vi "activeXexample.vi"() -> ()   [LabVIEW 2017]
panel:
  out "ID":i32
  out "Acq":i32
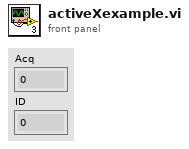
[diagram p1: front panel]
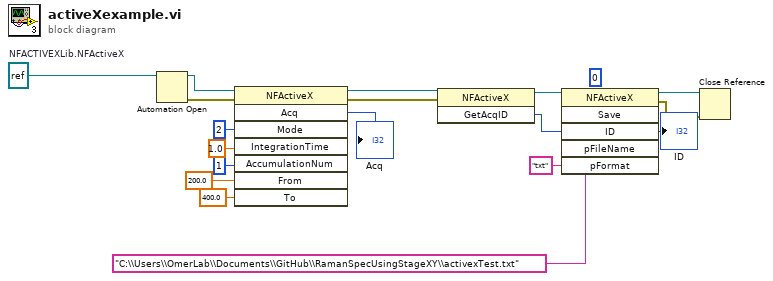
[diagram p0: block diagram]
diagram:
  (unwired) 0 ("Save")
  w16 = refnum<k7> refnum  # NFACTIVEXLib.NFActiveX
  n1 = Automation Open(Automation Refnum=w16) -> (Automation Refnum=w18:refnum<k7>, error out=w17:errorcluster)  [unwired: 3 in]
  n2 = invoke class="NFActiveX" method="Acq"(reference=w18, error in=w17, "Mode"=2, "IntegrationTime"=1.0, "AccumulationNum"=1, "From"=200.0, "To"=400.0) -> (reference out=w9:refnum<k7>, error out=w8:errorcluster, "Acq"=→"Acq":i32)  [unwired: 1 in, 5 out]
  n3 = invoke class="NFActiveX" method="GetAcqID"(reference=w9, error in=w8) -> (reference out=w6:refnum<k7>, "GetAcqID"=w7:i32)  [unwired: 1 in, 1 out]
  n4 = invoke class="NFActiveX" method="Save"(reference=w6, "ID"=w7, "pFileName"="C:\\Users\\OmerLab\\Documents\\GitHub\\RamanSpecUsingStageXY\\activexTest.txt", "pFormat"="txt") -> (reference out=w4:refnum<k7>, error out=w3:errorcluster, "ID"=→"ID":i32)  [unwired: 2 in, 3 out]
  n5 = Close Reference(reference=w4, error in (no error)=w3) -> ()  [unwired: 1 out]
